vi "HandleDrive.vi"(7 "Sensitivity":dbl=0.01, 8 "StraightDrive":bool, 9 "HalfDrive":bool, 10 "RightMotor":dbl, 11 "LeftMotor":dbl) -> (3 "Enqueue?":bool)   [LabVIEW 2013]
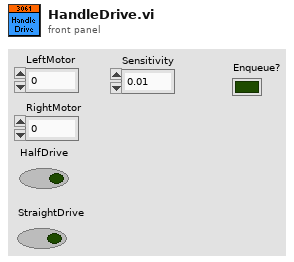
[diagram p1: front panel]
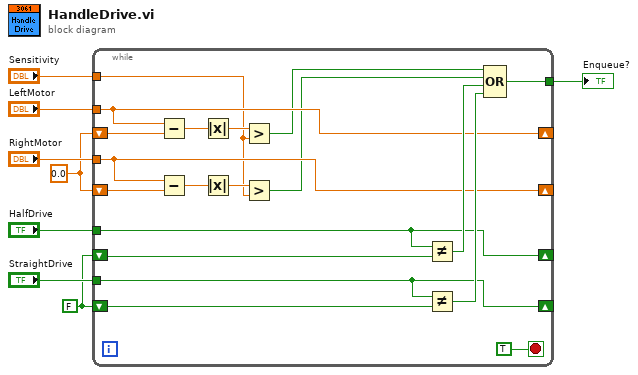
[diagram p0: block diagram]
diagram:
  w2 = 0.0 ("LeftMotor")
  w4 = FALSE ("HalfDrive")
  n1 = while {
    tunnel: "HalfDrive" -> [w20]
    tunnel: "LeftMotor" -> [w12]
    tunnel: "RightMotor" -> [w17]
    tunnel: "StraightDrive" -> [w19]
    shift-right: [w20] -> _
    shift-left: w4 -> [w21]
    shift-right: [w19] -> _
    shift-left: w4 -> [w22]
    shift-right: [w12] -> _
    shift-left: w2 -> [w13]
    shift-right: [w17] -> _
    shift-left: w2 -> [w18]
    tunnel: [w24] -> w3
    tunnel: "Sensitivity" -> [w11]
    stop <- TRUE stop-if-true
    n2 = Subtract(x=w12, y=w13) -> (x-y=w15:dbl)
    n3 = Subtract(x=w17, y=w18) -> (x-y=w23:dbl)
    n4 = Absolute Value(x=w15) -> (abs(x)=w14:dbl)
    n5 = Absolute Value(x=w23) -> (abs(x)=w16:dbl)
    n6 = Greater?(x=w14, y=w11) -> (0:w10:bool)
    n7 = Greater?(x=w16, y=w11) -> (0:w9:bool)
    n8 = Not Equal?(x=w20, y=w21) -> (x != y?=w25:bool)
    n9 = Not Equal?(x=w19, y=w22) -> (x != y?=w26:bool)
    n10 = Compound Arithmetic op=OR(w10, w9, w25, w26) -> (w24:bool)
  }
  "Enqueue?" <- w3
